vi "Init_LoG_Settings-1.vi"(0 "Dim #1":u8, 1 "Sigma #1":dbl, 2 "Expanding Factor":u16, 3 "Dim #2":u8, 4 "Sigma #2":dbl) -> (6 "LoG Settings":T1)   [LabVIEW 2013]
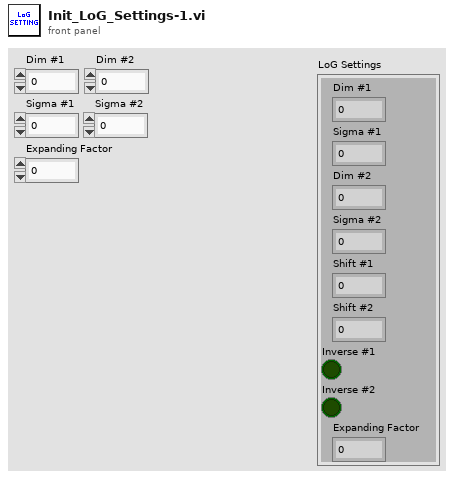
[diagram p1: front panel]
types:
  T1 = cluster{"Dim #1":u8, "Sigma #1":dbl, "Dim #2":u8, "Sigma #2":dbl, "Shift #1":u16, "Shift #2":u16, "Inverse #1":bool, "Inverse #2":bool, "Expanding Factor":u16}
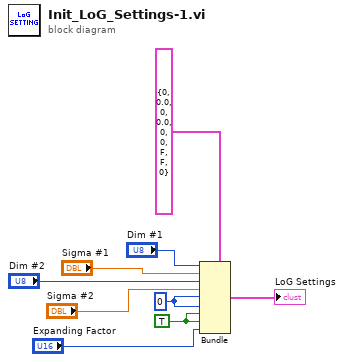
[diagram p0: block diagram]
diagram:
  w7 = TRUE
  w6 = u16 0 ("Shift")
  n1 = Bundle(cluster=T1 {"Dim #1"=0, "Sigma #1"=0.0, "Dim #2"=0, "Sigma #2"=0.0, "Shift #1"=0, "Shift #2"=0, "Inverse #1"=FALSE, "Inverse #2"=FALSE, "Expanding Factor"=0}, "Dim #1"="Dim #1", "Sigma #1"="Sigma #1", "Dim #2"="Dim #2", "Sigma #2"="Sigma #2", "Shift #1"=w6, "Shift #2"=w6, "Inverse #1"=w7, "Inverse #2"=w7, "Expanding Factor"="Expanding Factor") -> (→"LoG Settings":T1)
